vi "TDMS.HandlePass.vi"(8 "error in (no error)":errorcluster, 11 "file path in":path) -> (0 "error out":errorcluster)   [LabVIEW 2014, in "NIAnalysis.lvlib"]
uses:
  NIAnalysis.lvlib
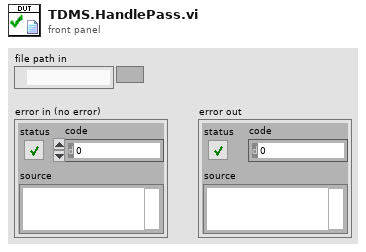
[diagram p1: front panel]
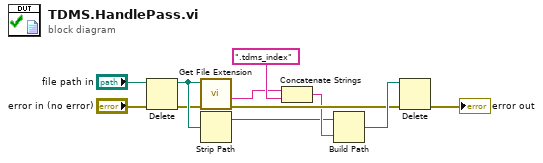
[diagram p0: block diagram]
diagram:
  n1 = Delete(path (use dialog)="file path in", error in="error in (no error)") -> (deleted path=w4:path, error out=w2:errorcluster)  [unwired: 3 in, 1 out]
  n2 = call <vilib>:"Get File Extension.vi"("error in (no error)"=w2, "file"=w4) -> ("error out"=w9:errorcluster, "filename without extension"=w6:string)  [unwired: 6 in, 2 out]
  n3 = Strip Path(path=w4) -> (stripped path=w5:path)  [unwired: 1 out]
  n4 = Concatenate Strings(w6, ".tdms_index" ("filename without extension")) -> (w8:string)
  n5 = Build Path(base path=w5, name or relative path=w8) -> (appended path=w11:path)
  n6 = Delete(path (use dialog)=w11, error in=w9) -> (error out=→"error out":errorcluster)  [unwired: 3 in, 2 out]
